vi "Wait on Rising Edge.vi"(11 "Refnum in":refnum<k21>) -> ()   [LabVIEW 2018, in "MCP3008.lvlib"]
uses:
  MCP3008.lvlib
  <vilib>/rvi/Emulation/niFpgaGetClockAttributes.vi
  <vilib>/rvi/Emulation/niFpgaSctlEmulationGetInTimedLoop.vi
  <vilib>/rvi/Emulation/niFpgaEmulationReportErrorSimple.vi
  <vilib>/rvi/eio/common/nirviEmuTemplateMethod_errors.vi
  <vilib>/rvi/Emulation/niFpgaCriticalErrorInLSC.vi
  <vilib>/eio/EIONode/EIONode.xnode
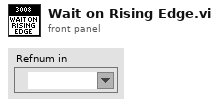
[diagram p1: front panel]
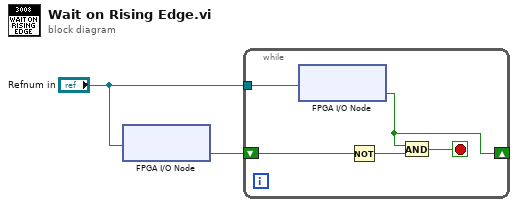
[diagram p0: block diagram]
diagram:
  n1 = xnode "FPGA I/O Node"("FPGA I/O In"="Refnum in") -> ("I/O Item"=w1:bool)  [unwired: 1 out]
  n2 = while {
    shift-right: [w5] -> _
    shift-left: w1 -> [w6]
    tunnel: "Refnum in" -> [w3]
    stop <- w4 stop-if-true
    n3 = xnode "FPGA I/O Node"("FPGA I/O In"=w3) -> ("I/O Item"=w5:bool)  [unwired: 1 out]
    n4 = Not(x=w6) -> (.not. x?=w7:bool)
    n5 = And(x=w5, y=w7) -> (x .and. y?=w4:bool)
  }
